vi "AddClassInline.vi"(9 "Count":i32, 11 "Math.lvclass":refnum<class "Math.lvclass">) -> (3 "Math.lvclass 2":refnum<class "Math.lvclass">)   [LabVIEW 2016, in "Math.lvclass"]
uses:
  Math.lvclass
  Math.lvclass/Math.ctl
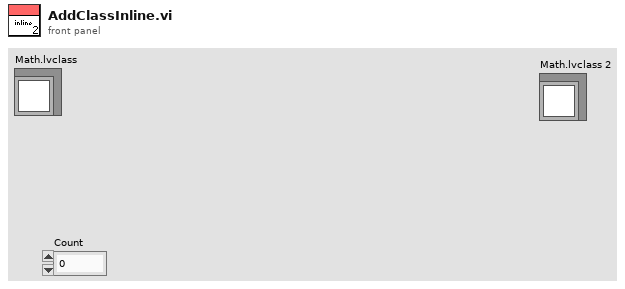
[diagram p1: front panel]
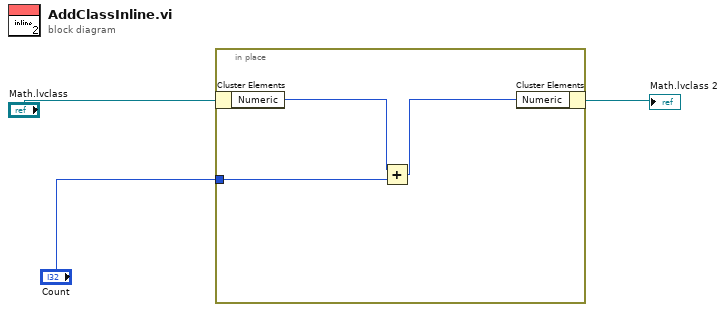
[diagram p0: block diagram]
diagram:
  n1 = in-place {
    in-place-border: "Count" -> [w6]
    n2 = in-place-cluster #1("Math.lvclass") -> ("Numeric"=w5:i32)
    n3 = Add(x=w5, y=w6) -> (x+y=w4:i32)
    n4 = in-place-cluster #1("Numeric"=w4) -> (→"Math.lvclass 2":refnum<class "Math.lvclass">)
  }
